vi "Test Create Logger with Rotating Daily File Sink.vi"(11 "Test Case In":refnum<class "Rotating Daily File Sink.lvclass">) -> (0 "error out":errorcluster, 3 "Test Case Out":refnum<class "Rotating Daily File Sink.lvclass">)   [LabVIEW 2020, in "Rotating Daily File Sink.lvclass"]
uses:
  Rotating Daily File Sink.lvclass
  C:/Program Files (x86)/National Instruments/LabVIEW 2020/vi.lib/Astemes/LUnit/Test Case.lvclass
  Source/Type Defs/Debug Level.ctl
  <vilib>/Astemes/LUnit/Test Case.lvclass/Test Case.ctl
  e0c7a7cc-5830-4673-a67d-18354674fd35.vi
  89f79ace-e66e-4d1c-86d9-b8788306fe36.vi
  8a204fe8-34b0-47c8-92ee-980a1ea9d0a5.vi
  <vilib>/Astemes/LUnit/Core/LUnit Test Case/Private/Append Fail Result.vi
  <vilib>/Astemes/LUnit/Core/LUnit Test Case/Private/Append Pass Result.vi
  e0c7a7cc-5830-4673-a67d-18354674fd35.vi/9c5d11cd-9439-4240-a1ee-d9baace9c924.vi
  89f79ace-e66e-4d1c-86d9-b8788306fe36.vi/9c5d11cd-9439-4240-a1ee-d9baace9c924.vi
  8a204fe8-34b0-47c8-92ee-980a1ea9d0a5.vi/9c5d11cd-9439-4240-a1ee-d9baace9c924.vi
  <vilib>/Astemes/LUnit/Core/LUnit Test Case/Private/Run In UI.vi
  <vilib>/Utility/error.llb/Clear Errors.vi
  Source/Sinks/Rotating File Sink/Rotating Daily File Sink.lvclass
  C:/Users/hughe_cx/Documents/05_repos/LVLog/Source/Sinks/Sink/Sink.lvclass
  Source/LV Log.lvlib
  Source/Logger/Logger.lvclass
  <vilib>/Astemes/LUnit/Test Case.lvclass
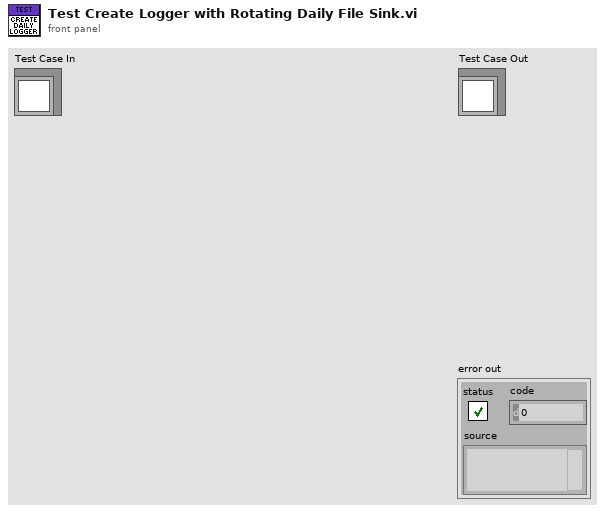
[diagram p1: front panel]
types:
  T1 = typedef "LV Log.lvlib/Debug Level.ctl" = enum16{"DEFAULT", "DEBUG", "INFO", "WARN", "ERROR", "FATAL"}
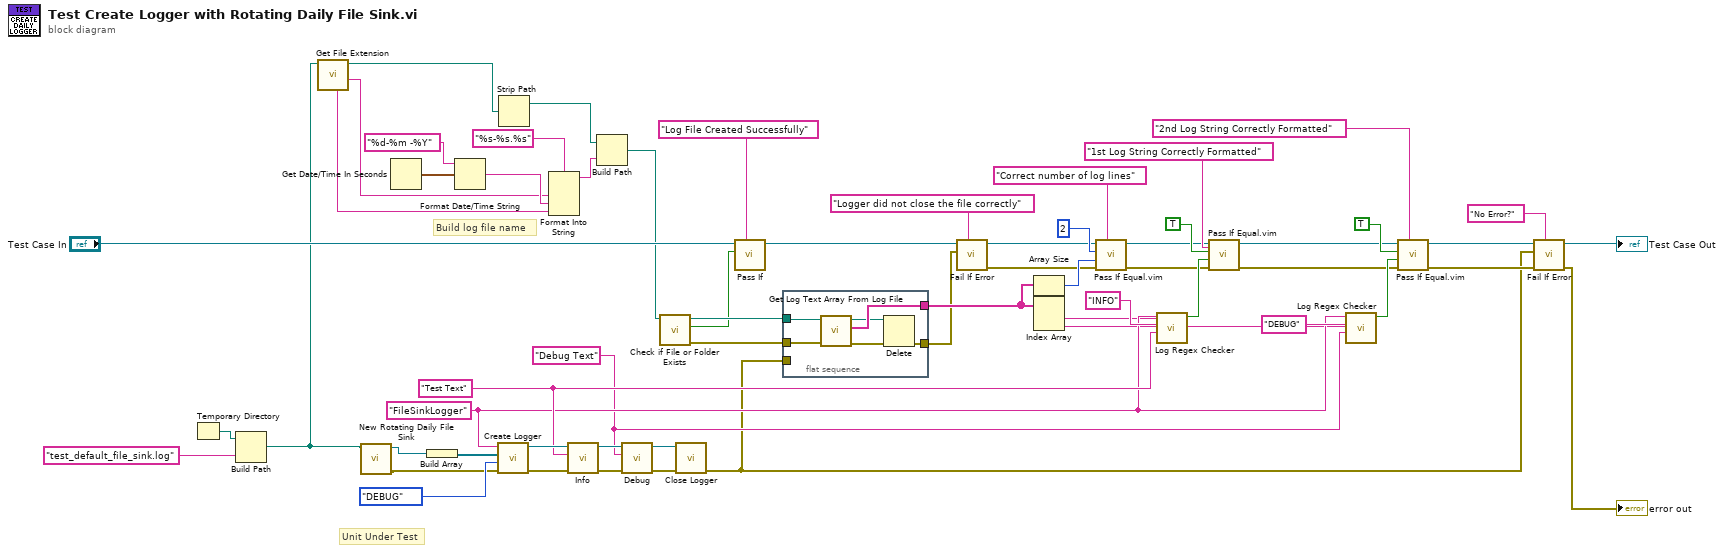
[diagram p0: block diagram]
diagram:
  w46 = "Debug Text" ("Log Text")
  w55 = "Test Text" ("Log Text")
  w47 = "FileSinkLogger" ("Name")
  # "Build log file name"
  # "Unit Under Test"
  n1 = Temporary Directory() -> (w60:path)
  n2 = Build Path(base path=w60, name or relative path="test_default_file_sink.log" ("format string")) -> (appended path=w3:path)
  n3 = call <vilib>:"Get File Extension.vi"("file"=w3) -> ("filename without extension"=w5:string, "dup file"=w1:path, "unmodified file extension"=w6:string)  [unwired: 6 in, 2 out]
  n4 = call "New Rotating Daily File Sink.vi"("File Path"=w3) -> ("error out"=w14:errorcluster, "Rotating Daily File Sink out"=w13:refnum<class "Rotating Daily File Sink.lvclass">)  [unwired: 9 in]
  n5 = Get Date/Time In Seconds() -> (seconds since 1Jan1904=w9:timestamp)
  n6 = Build Array(w13) -> (w30:refnum<class "Rotating Daily File Sink.lvclass">[])
  n7 = Format Date/Time String(time format string (%c)="%d-%m -%Y", seconds (now)=w9) -> (date/time string=w10:string)  [unwired: 1 in]
  n8 = call "Create Logger.vi"("error in (no error)"=w14, "Debug Level (Default)"=Debug_Level."DEBUG" ("Debug Level in"), "Sinks (Default)"=w30, "Name"=w47) -> ("error out"=w59:errorcluster, "Logger out"=w58:refnum<class "Logger.lvclass">)  [unwired: 6 in]
  n9 = Strip Path(path=w1) -> (stripped path=w7:path)  [unwired: 1 out]
  n10 = Format Into String(format string="%s-%s.%s", w5, w10, w6) -> (resulting string=w8:string)  [unwired: 2 in, 1 out]
  n11 = call "Info.vi"("error in (no error)"=w59, "Log Text"=w55, "Logger in"=w58) -> ("error out"=w54:errorcluster, "Logger out"=w53:refnum<class "Logger.lvclass">)  [unwired: 6 in, 1 out]
  n12 = Build Path(base path=w7, name or relative path=w8) -> (appended path=w2:path)
  n13 = call "Debug.vi"("error in (no error)"=w54, "Log Text"=w46, "Logger in"=w53) -> ("error out"=w28:errorcluster, "Logger out"=w27:refnum<class "Logger.lvclass">)  [unwired: 6 in, 1 out]
  n14 = call <vilib>:"Check if File or Folder Exists.vi"("path"=w2) -> ("error out"=w33:errorcluster, "file or folder exists?"=w32:bool, "dup path"=w34:path)  [unwired: 8 in]
  n15 = call "Close Logger.vi"("error in (no error)"=w28, "Logger in"=w27) -> ("error out"=w26:errorcluster)  [unwired: 9 in]
  n16 = call <vilib>:"Pass If.vi"("Description"="Log File Created Successfully", "Pass?"=w32, "LUnit Test Case In"="Test Case In") -> ("LUnit Test Case Out"=w23:refnum<class "Rotating Daily File Sink.lvclass">)  [unwired: 7 in, 1 out]
  n17 = flat-sequence {
    tunnel: w34 -> [w66]
    tunnel: [w65] -> w40
    tunnel: w33 -> [w62]
    tunnel: w26 -> [_]
    tunnel: [w61] -> w19
    frame #0 {
      n18 = call "Get Log Text Array From Log File.vi"("error in"=w62, "Log File Path in"=w66) -> ("error out"=w64:errorcluster, "Log Text Array"=w65:string[], "Log File Path out"=w63:path)  [unwired: 7 in]
      n19 = Delete(path (use dialog)=w63, error in=w64) -> (error out=w61:errorcluster)  [unwired: 3 in, 2 out]
    }
  }
  n20 = call <vilib>:"Fail If Error.vi"("Description"="Logger did not close the file correctly", "Assert error"=w19, "LUnit Test Case In"=w23) -> ("error out"=w20:errorcluster, "LUnit Test Case Out"=w22:refnum<class "Rotating Daily File Sink.lvclass">)  [unwired: 7 in]
  n21 = Array Size(array=w40) -> (size(s)=w39:i32)
  n22 = Index Array(array=w40) -> (element #1=w45:string, element #2=w44:string)  [unwired: 2 in]
  n23 = call "Pass If Equal.vim"("Description"="Correct number of log lines", "error in (no error)"=w20, "Actual"=w39, "Expected"=2, "LUnit Test Case In"=w22) -> ("error out"=w35:errorcluster, "LUnit Test Case Out"=w41:refnum<class "Rotating Daily File Sink.lvclass">)  [unwired: 5 in]
  n24 = call "Log Regex Checker.vi"("Log String"=w45, "Expected Log Text (Any)"=w55, "Expected Log Level (Any)"="INFO", "Expected Logger Name (Any)"=w47) -> ("Math Found"=w51:bool)  [unwired: 5 in, 2 out]
  n25 = call "Pass If Equal.vim"("Description"="1st Log String Correctly Formatted", "error in (no error)"=w35, "Actual"=w51, "Expected"=TRUE, "LUnit Test Case In"=w41) -> ("error out"=w36:errorcluster, "LUnit Test Case Out"=w43:refnum<class "Rotating Daily File Sink.lvclass">)  [unwired: 5 in]
  n26 = call "Log Regex Checker.vi"("Log String"=w44, "Expected Log Text (Any)"=w46, "Expected Log Level (Any)"="DEBUG", "Expected Logger Name (Any)"=w47) -> ("Math Found"=w50:bool)  [unwired: 5 in, 2 out]
  n27 = call "Pass If Equal.vim"("Description"="2nd Log String Correctly Formatted", "error in (no error)"=w36, "Actual"=w50, "Expected"=TRUE, "LUnit Test Case In"=w43) -> ("error out"=w37:errorcluster, "LUnit Test Case Out"=w42:refnum<class "Rotating Daily File Sink.lvclass">)  [unwired: 5 in]
  n28 = call <vilib>:"Fail If Error.vi"("Description"="No Error?", "error in (no error)"=w37, "Assert error"=w26, "LUnit Test Case In"=w42) -> ("error out"=→"error out":errorcluster, "LUnit Test Case Out"=→"Test Case Out":refnum<class "Rotating Daily File Sink.lvclass">)  [unwired: 6 in]
